vi "ThrustDataCollection.vi"() -> ()   [LabVIEW 2022 SP3]
uses:
  <vilib>/Analysis/NI_AALBase.lvlib
  STOP_GLOBAL.vi
  <vilib>/Analysis/baseanly.llb/Mean (DBL).vi
panel:
  in  "Tab Control":enum32{"Test Firing", "Non_Important"}(tab)
  out "Thrust Data 2":dbl[](graph)
  out "Thrust Data":dynamicdata(graph)
  out "Thrust Data 3":dbl[](graph)
  out "Thrust Data 4":dynamicdata(graph)
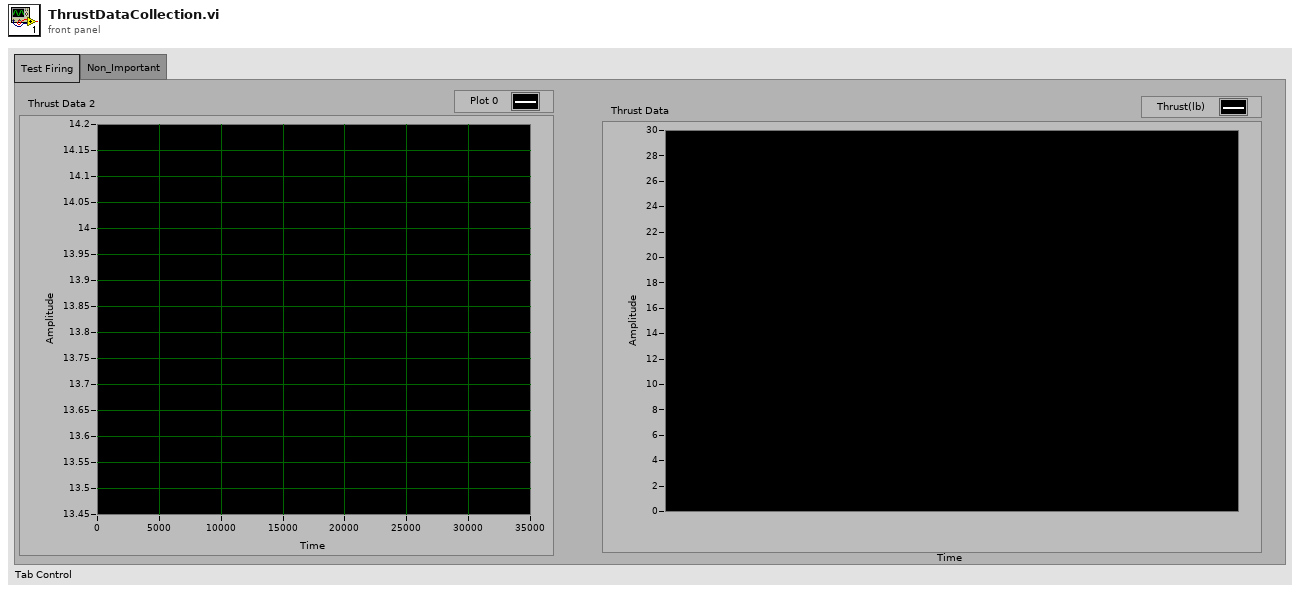
[diagram p1: front panel]
types:
  T1 = enum16{"Left Button", "Center Button", "Right Button", "Window Close"}
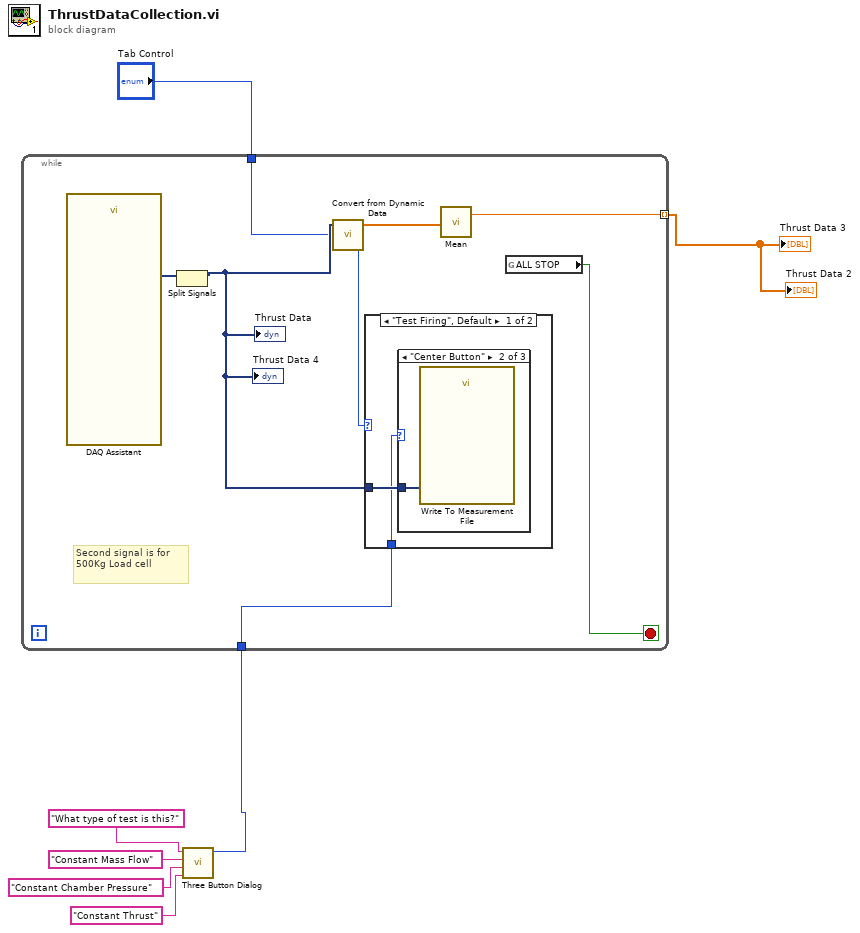
[diagram p0: block diagram]
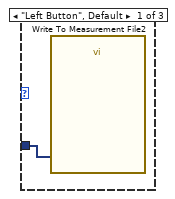
[diagram p2: hidden frame]
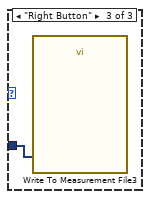
[diagram p3: hidden frame]
diagram:
  n1 = call <vilib>:"Three Button Dialog.vi"("Right Button Text (\"Cancel\")"="Constant Thrust" ("Right Button Text (\"Cancel\")"), "Center Button Text (\"No\")"="Constant Chamber Pressure" ("Center Button Text (\"No\")"), "Left Button Text (\"Yes\")"="Constant Mass Flow" ("Left Button Text (\"Yes\")"), "message"="What type of test is this?") -> ("Which Button?"=w2:T1)  [unwired: 7 in]
  n2 = while {
    tunnel: "Tab Control" -> [w11]
    tunnel: w2 -> [w10]
    tunnel: [w8] -> w1 mode=indexing
    stop <- w9 stop-if-true
    # "Second signal is for 500Kg Load cell"
    n3 = call "DAQ Assistant"() -> ("data"=w14:dynamicdata)  [unwired: 16 in, 3 out]
    n4 = Split Signals(w14) -> (w13:dynamicdata)  [unwired: 2 in, 1 out]
    "Thrust Data" <- w13
    "Thrust Data 4" <- w13
    n5 = call "Convert from Dynamic Data"("Dynamic Data Type"=w13) -> ("Array"=w12:dbl[])  [unwired: 3 in]
    n6 = case shown="\"Test Firing\", Default" w11 {
      tunnel: w13 -> [w16 _]
      tunnel: w10 -> [w15 _]
      frame "Test Firing", Default {
        n7 = case shown="\"Center Button\"" w15 {
          tunnel: w16 -> [w17 w18 w19]
          frame "Left Button", Default {
            n8 = call "Write To Measurement File2"("Signals"=w17) -> ()  [unwired: 16 in, 3 out]
          }
          frame "Center Button" {
            n9 = call "Write To Measurement File"("Signals"=w18) -> ()  [unwired: 16 in, 3 out]
          }
          frame "Right Button" {
            n10 = call "Write To Measurement File3"("Signals"=w19) -> ()  [unwired: 16 in, 3 out]
          }
        }
      }
      frame "Non_Important" {
      }
    }
    n11 = call-poly <vilib>:"Mean.vi"("X"=w12) -> ("mean"=w8:dbl)  [unwired: 1 out]
    n12 = global read "STOP_GLOBAL.vi" "ALL STOP"() -> (w9:bool)
  }
  "Thrust Data 2" <- w1
  "Thrust Data 3" <- w1
